vi "Translation3d_Interpolate.vi"(9 "T":dbl, 10 "other Translation3d":T1 {"Z" format="%14.3f"; "Y" format="%14.3f"; "X" format="%14.3f"}, 11 "In Translation3d":T1 {"Z" format="%14.3f"; "Y" format="%14.3f"; "X" format="%14.3f"}) -> (3 "Interpolated Translation3d":T1 {"Z" format="%14.3f"; "Y" format="%14.3f"; "X" format="%14.3f"})   [LabVIEW 2019, in "Trajectory_Library.lvlib"]
doc: "Inerpolate between this and an End Value translation\n \n\nParameters:\n - IN Translation - This translation data structure\n - EndValue Translation - The translation data structure\n\nReturns\n - Interpolated Translation - The interpolated translation."
uses:
  Trajectory_Library.lvlib
  TRANSLATION3D.ctl
  MathUtil_Clamp.vi
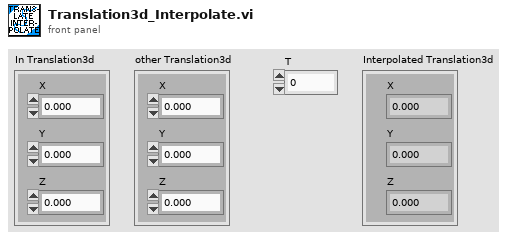
[diagram p1: front panel]
types:
  T1 = typedef "Trajectory_Library.lvlib/TRANSLATION3D.ctl" = cluster{"X":dbl, "Y":dbl, "Z":dbl}
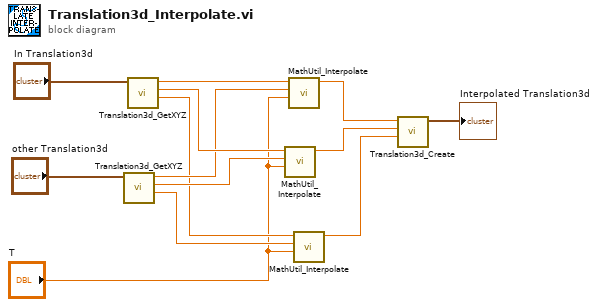
[diagram p0: block diagram]
diagram:
  n1 = call "Translation3d_GetXYZ.vi"("In Translation3d"="other Translation3d") -> ("Z"=w3:dbl, "Y"=w6:dbl, "X"=w7:dbl)  [unwired: 8 in]
  n2 = call "Translation3d_GetXYZ.vi"("In Translation3d"="In Translation3d") -> ("Z"=w4:dbl, "Y"=w9:dbl, "X"=w10:dbl)  [unwired: 8 in]
  n3 = call "MathUtil_Interpolate.vi"("T"="T", "EndValue"=w6, "StartValue"=w9) -> ("InterpolatedValue"=w11:dbl)  [unwired: 8 in]
  n4 = call "MathUtil_Interpolate.vi"("T"="T", "EndValue"=w7, "StartValue"=w10) -> ("InterpolatedValue"=w12:dbl)  [unwired: 8 in]
  n5 = call "MathUtil_Interpolate.vi"("T"="T", "EndValue"=w3, "StartValue"=w4) -> ("InterpolatedValue"=w1:dbl)  [unwired: 8 in]
  n6 = call "Translation3d_Create.vi"("Z"=w1, "Y"=w11, "X"=w12) -> ("TRANSLATION3D"=→"Interpolated Translation3d":T1)  [unwired: 8 in]
